vi "ACQ Rozdziel kanaly analogowe.vi"(8 "error in (no error)":errorcluster, 10 "Kanaly in":T1, 11 "data":waveform(dbl)[](array[waveform])) -> (0 "error out":errorcluster, 2 "Kanaly out":T1)   [LabVIEW 2013]
doc: "Rozdziela kanały z wejść analogowych karty na:\nanalogowe, cyfrowe, zwarcie."
uses:
  Kontrolki/Przetwarzanie/Kanaly.ctl
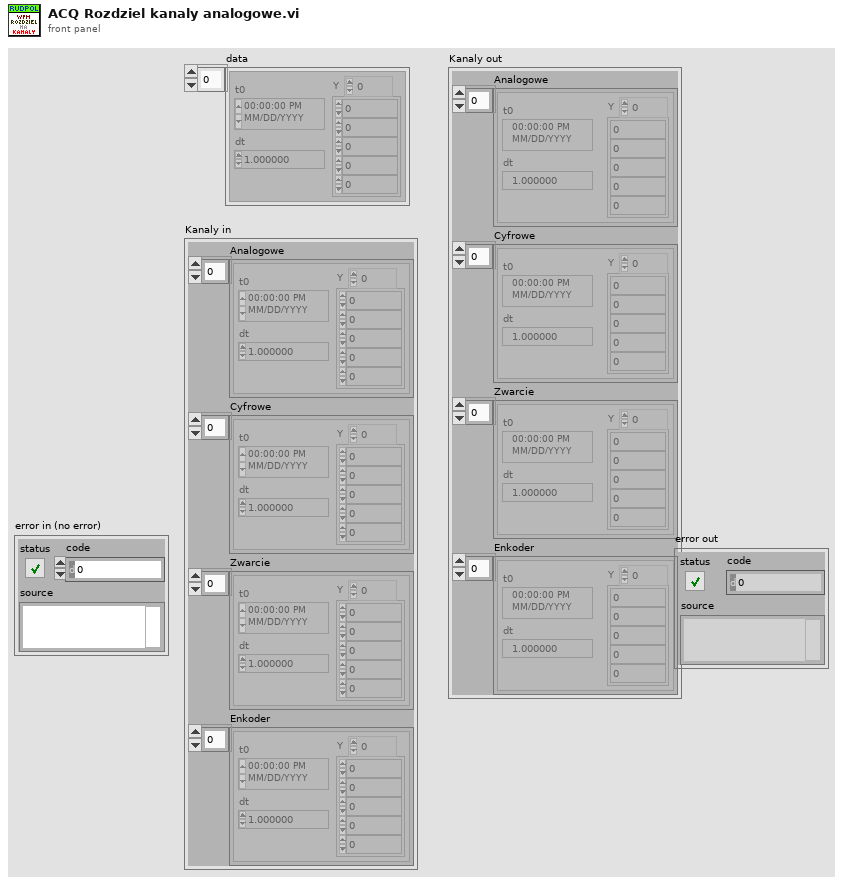
[diagram p1: front panel]
types:
  T1 = typedef "Kanaly.ctl" = cluster{"Analogowe":waveform(dbl)[], "Cyfrowe":waveform(dbl)[], "Zwarcie":waveform(dbl)[], "Enkoder":waveform(dbl)[]}
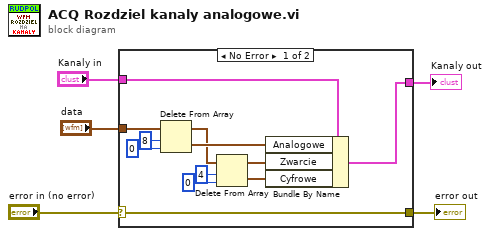
[diagram p0: block diagram]
diagram:
  n1 = case shown="No Error" "error in (no error)" {
    selector: "error in (no error)" -> [w6 w18]
    tunnel: [w17 w19] -> w5
    tunnel: "Kanaly in" -> [w13 w19]
    tunnel: "data" -> [w7 _]
    tunnel: [w6 w18] -> w1
    frame No Error {
      n2 = Delete From Array(array=w7, length=8, index=0) -> (deleted portion=w14:waveform(dbl)[], array with subset deleted=w8:waveform(dbl)[])
      n3 = Delete From Array(array=w8, length=4, index=0) -> (deleted portion=w15:waveform(dbl)[], array with subset deleted=w16:waveform(dbl)[])
      n4 = Bundle By Name(cluster=w13, "Analogowe"=w14, "Zwarcie"=w16, "Cyfrowe"=w15) -> (w17:T1)
    }
    frame Error {
    }
  }
  "Kanaly out" <- w5
  "error out" <- w1
